vi "database.vi"   [LabVIEW 2017]
uses:
  <vilib>/drjdpowell/SQLite Library/SQL Statement/SQL Statement.lvclass/SQL Statement.ctl
  <vilib>/drjdpowell/SQLite Library/SQL Connection/Open (path).vi
  <vilib>/drjdpowell/SQLite Library/SQL Statement/Bind Real.vi
  <vilib>/drjdpowell/SQLite Library/SQL Connection/Open (string).vi
  <vilib>/drjdpowell/SQLite Library/SQL Statement/Step.vi
  <vilib>/AdvancedString/Path To Command Line String.vi
  <vilib>/drjdpowell/SQLite Library/SQL Connection/Execute SQL (No results).vi
  <vilib>/drjdpowell/SQLite Library/SQL Statement/Error Message.vi
  <vilib>/drjdpowell/SQLite Library/SQL Connection/Connection.lvclass
  <vilib>/drjdpowell/SQLite Library/SQL Statement/SQL Statement.lvclass
  <vilib>/drjdpowell/SQLite Library/Transaction Helpers/Transaction.lvlib
  <vilib>/drjdpowell/SQLite Library/SQLite.lvlib
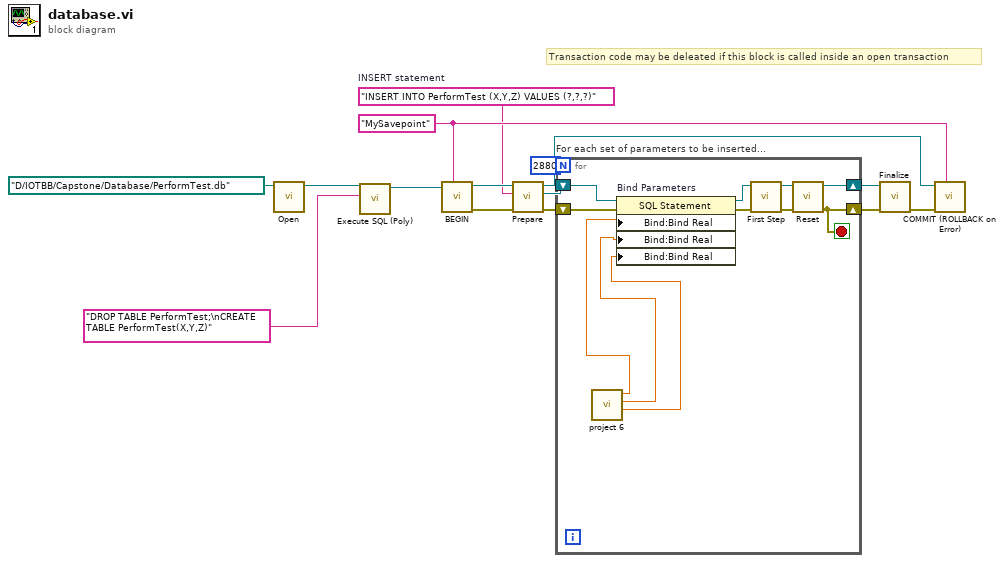
[diagram p0: block diagram]
diagram:
  w11 = "MySavepoint" ("Savepoint name")
  w6 = "INSERT INTO PerformTest (X,Y,Z) VALUES (?,?,?)"  # INSERT statement
  # "Transaction code may be deleated if this block is called inside an open transaction"
  n1 = call-poly <vilib>:"Open.vi"("db file"=path "D:/IOTBB/Capstone/Database/PerformTest.db") -> ("SQLite Connection"=w15:refnum<class "Connection.lvclass">)  [unwired: 9 in, 1 out]
  n2 = call-poly <vilib>:"Execute SQL (Poly).vi"("SQL"="DROP TABLE PerformTest;\nCREATE TABLE PerformTest(X,Y,Z)", "SQLite Connection in"=w15) -> ("SQLite Connection"=w3:refnum<class "Connection.lvclass">)  [unwired: 8 in, 1 out]
  n3 = call <vilib>:"BEGIN.vi"("Savepoint name"=w11, "Connection in"=w3) -> ("error out"=w10:errorcluster, "Connection out"=w9:refnum<class "Connection.lvclass">)  [unwired: 8 in]
  n4 = call <vilib>:"Prepare.vi"("error in (no error)"=w10, "SQL"=w6, "SQLite Connection in"=w9) -> ("error out"=w5:errorcluster, "SQL Statement"=w4:refnum<class "SQL Statement.lvclass">, "SQLite Connection"=w12:refnum<class "Connection.lvclass">)  [unwired: 4 in, 2 out]
  n5 = for "For each set of parameters to be inserted..." {
    N: 2880 -> [_]
    shift-right: [w20] -> w7
    shift-left: w4 -> [w26]
    shift-right: [w19] -> w8
    shift-left: w5 -> [w23]
    stop <- w19 stop-if-true
    n6 = call "project 6.vi"() -> ("Fail"=w16:dbl, "Pass"=w17:dbl, "Total"=w18:dbl)  [unwired: 9 in]
    n7 = property on="Bind Parameters" class="SQL Statement"(reference=w26, error in=w23, "Bind:Bind Real"=w18, "Bind:Bind Real"=w17, "Bind:Bind Real"=w16) -> (reference out=w25:refnum<class "SQL Statement.lvclass">, error out=w24:errorcluster)
    n8 = call <vilib>:"First Step.vi"("error in (no error)"=w24, "SQL Statement in"=w25) -> ("error out"=w22:errorcluster, "SQL Statement"=w21:refnum<class "SQL Statement.lvclass">)  [unwired: 7 in, 1 out]
    n9 = call <vilib>:"Reset.vi"("error in (no error)"=w22, "SQL Statement in"=w21) -> ("error out"=w19:errorcluster, "SQL Statement"=w20:refnum<class "SQL Statement.lvclass">)  [unwired: 8 in]
  }
  n10 = call <vilib>:"Finalize.vi"("error in (no error)"=w8, "SQL Statement in"=w7) -> ("error out"=w13:errorcluster)  [unwired: 9 in]
  n11 = call <vilib>:"COMMIT (ROLLBACK on Error).vi"("Savepoint name"=w11, "error in (no error)"=w13, "Connection in"=w12) -> ()  [unwired: 7 in, 2 out]
